vi "Read From String Delimiter.vi"(8 "error in (no error)":errorcluster, 11 "Abs_Value_1D in":refnum<class "Abs_Value_1D.lvclass">) -> (0 "error out":errorcluster, 2 "Delimiter":string, 3 "Abs_Value_1D out":refnum<class "Abs_Value_1D.lvclass">)   [LabVIEW 2021, in "Abs_Value_1D.lvclass"]
uses:
  Abs_Value_1D.lvclass
  Abs_Value_1D.lvclass/Abs_Value_1D.ctl
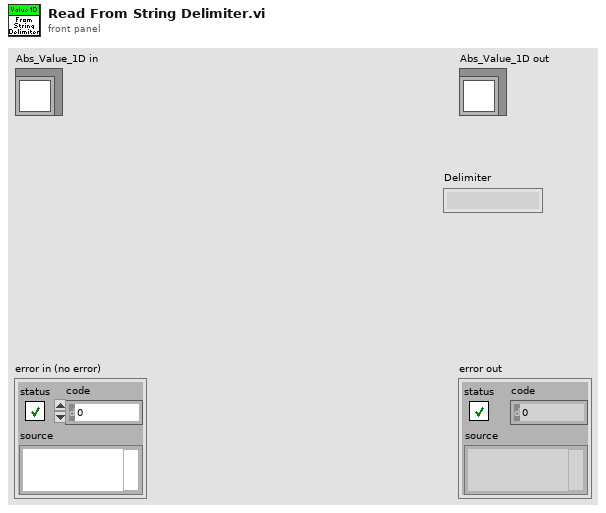
[diagram p1: front panel]
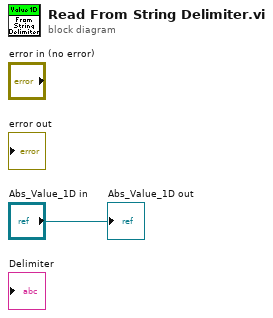
[diagram p0: block diagram]
diagram:
  "Abs_Value_1D out" <- "Abs_Value_1D in"
